vi "WriteUncTURReport.vi"(8 "error in (no error)":errorcluster, 10 "TUR":dbl[][][](array[numeric]), 11 "UNC":dbl[][][](array[numeric])) -> (0 "error out":errorcluster)   [LabVIEW 2014]
uses:
  Excel(ActiveX)/enumOpenOrCreate.ctl
  Excel(ActiveX)/Excel(ActiveX).lvlib
panel:
  in  "Row Labels":string[](array[string])=["VA", "VB", "VC", "V+", "IA", "IB", "IC", "I+", "Freq", "ROCOF"]
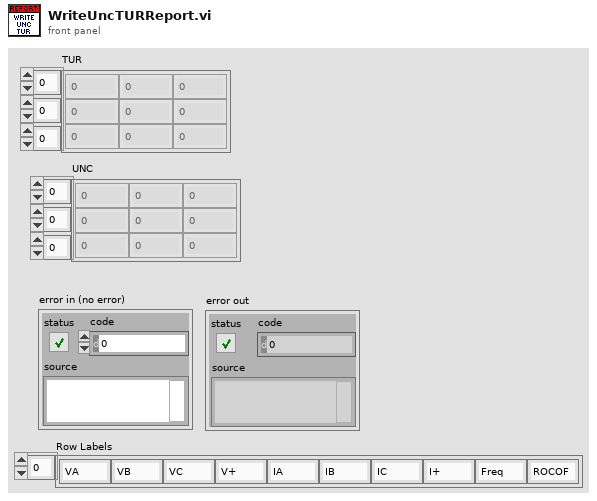
[diagram p1: front panel]
types:
  T1 = typedef "Excel(ActiveX).lvlib/enumOpenOrCreate.ctl" = enum16{"open", "open or create", "create from template"}
  T2 = typedef "Excel(ActiveX).lvlib/ExcelActiveX.ctl" = cluster{"Excel._Application":refnum<k7>, "Application open at start":bool, "Excel._Worksheet":refnum<k7>, "Workbook open at start":bool, "Excel._Workbook":refnum<k7>, "Workbook Path":path, "Worksheet Name":string, "Row":u32, "Col":u32, "Cell":string, "Workbook Name":string}
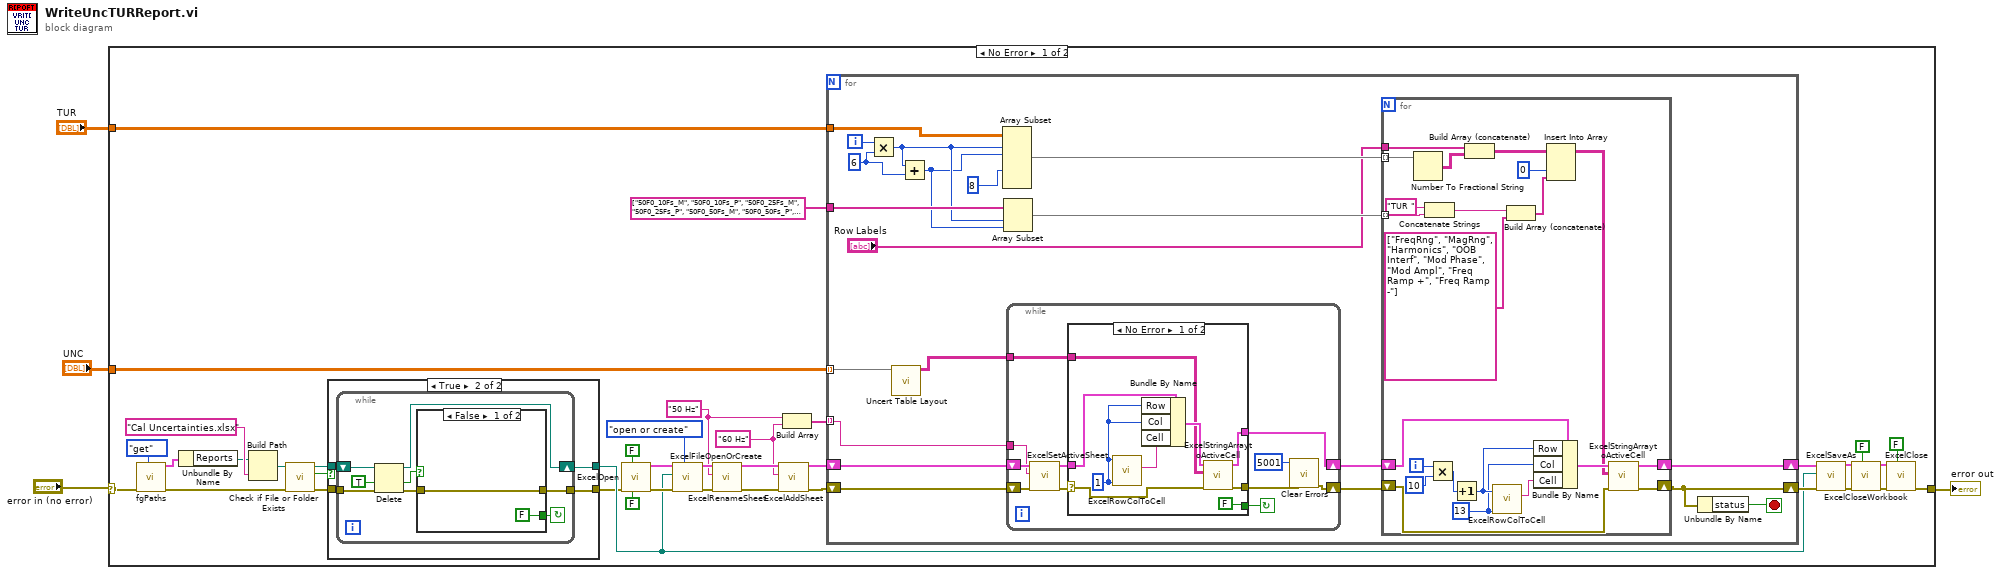
[diagram p0: block diagram]
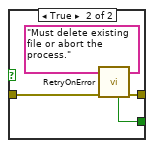
[diagram p3: hidden frame]
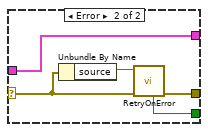
[diagram p4: hidden frame]
diagram:
  n1 = case shown="No Error" "error in (no error)" {
    selector: "error in (no error)" -> [w40 w130]
    tunnel: [w17 w130] -> w3
    tunnel: "UNC" -> [w25 _]
    tunnel: "TUR" -> [w14 _]
    frame No Error {
      w15 = "60 Hz"
      w16 = "50 Hz"
      n2 = call "fgPaths.vi"("cmd"=enum16{"init", "set", "get"}."get", "error in (no error)"=w40) -> ("error out"=w11:errorcluster, "clPaths"=w38:cluster{"Templates":path, "Reports":path})  [unwired: 8 in]
      n3 = Unbundle By Name(w38) -> ("Reports"=w33:path)
      n4 = Build Path(base path=w33, name or relative path="Cal Uncertainties.xlsx") -> (appended path=w12:path)
      n5 = call <vilib>:"Check if File or Folder Exists.vi"("error in (no error)"=w11, "path"=w12) -> ("error out"=w8:errorcluster, "file or folder exists?"=w10:bool, "dup path"=w9:path)  [unwired: 7 in]
      n6 = case shown="True" w10 {
        tunnel: w9 -> [w43 w48]
        tunnel: w8 -> [w44 w47]
        tunnel: [w44 w45] -> w6
        tunnel: [w43 w46] -> w7
        frame False {
        }
        frame True {
          n7 = while {
            shift-right: [w53] -> w46
            shift-left: w48 -> [w55]
            tunnel: w47 -> [w54]
            tunnel: [w51] -> w45
            stop <- w49 continue-if-true
            n8 = Delete(path (use dialog)=w55, confirm (F)=TRUE, error in=w54) -> (deleted path=w53:path, cancelled=w50:bool, error out=w52:errorcluster)  [unwired: 2 in]
            n9 = case shown="False" w50 {
              tunnel: w52 -> [w58 w60]
              tunnel: [w58 w62] -> w51
              tunnel: [FALSE ("Retry") w61] -> w49
              frame False {
              }
              frame True {
                n10 = call "RetryOnError.vi"("error in (no error)"=w60, "Error Msg"="Must delete existing file or abort the process.") -> ("error out"=w62:errorcluster, "Retry"=w61:bool)  [unwired: 8 in]
              }
            }
          }
        }
      }
      n11 = call "ExcelOpen.vi"("Run Minimized (f)"=FALSE, "Excel visible? (t)"=FALSE, "error in (no error)"=w6) -> ("error out"=w37:errorcluster, "ExcelActiveX"=w35:T2)  [unwired: 7 in]
      n12 = call "ExcelFileOpenOrCreate.vi"("Open or Create"=enumOpenOrCreate."open or create", "error in (no error)"=w37, "Excel file name and path"=w7, "ExcelActiveX in"=w35) -> ("error out"=w32:errorcluster, "ExcelActiveX out"=w31:T2)  [unwired: 6 in]
      n13 = call "ExcelRenameSheet.vi"("error in (no error)"=w32, "Sheet Name"=w16, "ExcelActiveX"=w31) -> ("error out"=w30:errorcluster, "ExcelActiveX 2"=w27:T2)  [unwired: 7 in]
      n14 = call "ExcelAddSheet.vi"("error in (no error)"=w30, "Sheet Name"=w15, "ExcelActiveX"=w27) -> ("error out"=w29:errorcluster, "ExcelActiveX"=w28:T2)  [unwired: 7 in]
      n15 = Build Array(w16, w15) -> (w26:string[])
      n16 = for {
        shift-right: [w66] -> w18
        shift-left: w28 -> [w81]
        shift-right: [w67] -> w19
        shift-left: w29 -> [w82]
        tunnel: w26 -> [w79] mode=indexing
        tunnel: w25 -> [w64] mode=indexing
        tunnel: w14 -> [w78]
        tunnel: string[] ["50F0_10Fs_M", "50F0_10Fs_P", "50F0_25Fs_M", "50F0_25Fs_P", "50F0_50Fs_M", "50F0_50Fs_P", "60F0_10Fs_M", "60F0_10Fs_P", "60F0_12Fs_M", "60F0_12Fs_P", "60F0_15Fs_M", "60F0_15Fs_P", "60F0_20Fs_M", "60F0_20Fs_P", "60F0_30Fs_M", "60F0_30Fs_P", "60F0_60Fs_M", "60F0_60Fs_P"] -> [w76]
        i -> [w77]
        stop <- w80 stop-if-true
        w75 = 6 ("y")
        n17 = Multiply(x=w77, y=w75) -> (x*y=w74:i32)
        n18 = call "Uncert Table Layout.vi"("Uncert In"=w64) -> ("Uncert Table"=w63:string[][])  [unwired: 10 in]
        n19 = Add(x=w74, y=w75) -> (x+y=w73:i32)
        n20 = Array Subset(array=w78, index (dim 0)=w74, length (dim 0)=w73, length (dim 1)=8 ("length")) -> (w70:dbl[][][])  [unwired: 3 in]
        n21 = Array Subset(array=w76, index=w74, length=w73) -> (w69:string[])
        n22 = while {
          tunnel: w63 -> [w106]
          shift-right: [w108] -> w71
          shift-left: w82 -> [w115]
          shift-right: [w107] -> w72
          shift-left: w81 -> [w114]
          tunnel: w79 -> [w105]
          stop <- w111 continue-if-true
          n23 = call "ExcelSetActiveSheet.vi"("error in (no error)"=w115, "Sheet Name"=w105, "ExcelActiveX in"=w114) -> ("error out"=w112:errorcluster, "ExcelActiveX  out"=w113:T2)  [unwired: 7 in]
          n24 = case shown="No Error" w112 {
            selector: w112 -> [w120 w128]
            tunnel: w113 -> [w124 w126]
            tunnel: [w121 w127] -> w109
            tunnel: [w118 w126] -> w107
            tunnel: [FALSE ("Retry") w125] -> w111
            tunnel: w106 -> [w117 _]
            frame No Error {
              w122 = u32 1 ("col")
              n25 = call "ExcelRowColToCell.vi"("col"=w122, "row"=w122) -> ("cell"=w123:string)  [unwired: 9 in]
              n26 = Bundle By Name(cluster=w124, "Row"=w122, "Col"=w122, "Cell"=w123) -> (w119:T2)
              n27 = call "ExcelStringArraytoActiveCell.vi"("error in (no error)"=w120, "Array"=w117, "ExcelActiveX"=w119) -> ("error out"=w121:errorcluster, "ExcelActiveX"=w118:T2)  [unwired: 7 in]
            }
            frame Error {
              n28 = Unbundle By Name(w128) -> ("source"=w129:string)
              n29 = call "RetryOnError.vi"("error in (no error)"=w128, "Error Msg"=w129) -> ("error out"=w127:errorcluster, "Retry"=w125:bool)  [unwired: 8 in]
            }
          }
          n30 = call <vilib>:"Clear Errors.vi"("error in (no error)"=w109, "specific error code to clear (0: all)"=5001) -> ("error out"=w108:errorcluster)  [unwired: 4 in, 1 out]
        }
        n31 = for {
          tunnel: w70 -> [w104] mode=indexing
          tunnel: w69 -> [w101] mode=indexing
          tunnel: "Row Labels" -> [w102]
          shift-right: [w84] -> w67
          shift-left: w71 -> [w87]
          shift-right: [w83] -> w66
          shift-left: w72 -> [w91]
          i -> [w94]
          w89 = u32 13 ("col")
          n32 = Number To Fractional String(number=w104) -> (F-format string=w103:string[][])  [unwired: 3 in]
          n33 = Concatenate Strings("TUR " ("string"), w101) -> (w99:string)
          n34 = Multiply(x=w94, y=10) -> (x*y=w92:i32)
          n35 = Increment(x=w92) -> (x+1=w90:i32)
          n36 = Build Array (concatenate)(w102, w103) -> (w97:string[][])
          n37 = call "ExcelRowColToCell.vi"("col"=w89, "row"=w90) -> ("cell"=w88:string)  [unwired: 9 in]
          n38 = Build Array (concatenate)(w99, string[] ["FreqRng", "MagRng", "Harmonics", "OOB Interf", "Mod Phase", "Mod Ampl", "Freq Ramp +", "Freq Ramp -"]) -> (w96:string[])
          n39 = Bundle By Name(cluster=w91, "Row"=w90, "Col"=w89, "Cell"=w88) -> (w86:T2)
          n40 = Insert Into Array(array=w97, index (col)=0 ("disabled index (col)"), new element=w96) -> (w85:string[][])  [unwired: 1 in]
          n41 = call "ExcelStringArraytoActiveCell.vi"("error in (no error)"=w87, "Array"=w85, "ExcelActiveX"=w86) -> ("error out"=w84:errorcluster, "ExcelActiveX"=w83:T2)  [unwired: 7 in]
        }
        n42 = Unbundle By Name(w67) -> ("status"=w80:bool)
      }
      n43 = call "ExcelSaveAs.vi"("error in (no error)"=w19, "Path"=w7, "ExcelActiveX"=w18) -> ("error out"=w20:errorcluster, "ExcelActiveX"=w22:T2)  [unwired: 7 in]
      n44 = call "ExcelCloseWorkbook.vi"("Save"=FALSE, "error in (no error)"=w20, "ExcelActiveX"=w22) -> ("error out"=w21:errorcluster, "ExcelActiveX"=w23:T2)  [unwired: 7 in]
      n45 = call "ExcelClose.vi"("Leave Open (f)"=FALSE, "error in (no error)"=w21, "ExcelActiveX in"=w23) -> ("error out"=w17:errorcluster)  [unwired: 7 in, 1 out]
    }
    frame Error {
    }
  }
  "error out" <- w3
